vi "TSLIN_Trace monitoring.vi"(10 "Data":T1={"Communication message"={"Sender"="", "receiver"="", "message"="", "data"=variant}, "LIN_Data"={"DLL_PATH"=path "", "Channels used"=1, "Funtiontype"=0, "Rx/TX"=enum."Rx", "Read message type"=enum."Receive&send messages", "async&sync"=enum."async", "sync_sendTimeout"=0, "LIN_SendHead"={"ALINIdxchn"=0, "ALINId"=0, "ALINDLC"=0}, "LIN_Set"={"Hardware Type"=2, "Hardware Subtype"=enum."TC1016", "AHwChannel"=0, "AAppChannel"=19, "ABaudrateKbps"=19.2, "AProtocol"=2, "AldHW"=0}, "LIN_DATA"={"Data0"=0, "Data1"=0, "Data2"=0, "Data3"=0, "Data4"=0, "Data5"=0, "Data6"=0, "Data7"=0}, "LIN_Set_Array"=[], "LDF"={"LDF Path"=path "", "LDF loading channel"=0}, "Blf_Log"={"Blf_Log_PATH"=path ""}, "LIN Scheduling Table Array"=[], "REC_Channel"=0}, "LIN Data array"=[], "error in"={"status"=FALSE, "code"=0, "source"=""}, "REC_Channel"=0, "AsynCall?"=FALSE, "DataBase_array"=refnum} {"REC_Channel" items=["CHN1", "CHN2", "CHN3", "CHN4", "CHN5", "CHN6", "CHN7", "CHN8", "CHN9", "CHN10", "CHN11", "CHN12", "CHN13", "CHN14", "CHN15", "CHN16", "CHN17", "CHN18", "CHN19", "CHN20", "CHN21", "CHN22", "CHN23", "CHN24", "CHN25", "CHN26", "CHN27", "CHN28", "CHN29", "CHN30", "CHN31", "CHN32"]; "LIN_Data"."REC_Channel" items=["CHN1", "CHN2", "CHN3", "CHN4", "CHN5", "CHN6", "CHN7", "CHN8", "CHN9", "CHN10", "CHN11", "CHN12", "CHN13", "CHN14", "CHN15", "CHN16", "CHN17", "CHN18", "CHN19", "CHN20", "CHN21", "CHN22", "CHN23", "CHN24", "CHN25", "CHN26", "CHN27", "CHN28", "CHN29", "CHN30", "CHN31", "CHN32"]; "LIN_Data"."LIN Scheduling Table Array"."LIN_Transmit"."Channel" items=["CHN1", "CHN2", "CHN3", "CHN4", "CHN5", "CHN6", "CHN7", "CHN8", "CHN9", "CHN10", "CHN11", "CHN12", "CHN13", "CHN14", "CHN15", "CHN16", "CHN17", "CHN18", "CHN19", "CHN20", "CHN21", "CHN22", "CHN23", "CHN24", "CHN25", "CHN26", "CHN27", "CHN28", "CHN29", "CHN30", "CHN31", "CHN32"]; "LIN_Data"."LIN Scheduling Table Array"."LIN_Transmit"."ID" format="%.0x"; "LIN_Data"."LIN Scheduling Table Array"."LIN_Transmit"."DLC" format="%.0x"; "LIN_Data"."LIN Scheduling Table Array"."LIN_Transmit"."Set_node_funtiontype" items=["MasterNode", "SlaveNode", "MonitorNote"]; "LIN_Data"."LDF"."LDF loading channel" items=["CHN1", "CHN2", "CHN3", "CHN4", "CHN5", "CHN6", "CHN7", "CHN8", "CHN9", "CHN10", "CHN11", "CHN12", "CHN13", "CHN14", "CHN15", "CHN16", "CHN17", "CHN18", "CHN19", "CHN20", "CHN21", "CHN22", "CHN23", "CHN24", "CHN25", "CHN26", "CHN27", "CHN28", "CHN29", "CHN30", "CHN31", "CHN32"]; "LIN_Data"."LIN_Set_Array"."Set_node_funtiontype" items=["MasterNode", "SlaveNode", "MonitorNote"]; "LIN_Data"."LIN_Set_Array"."Set"."Hardware Type" items=["BUS_UNKNOWN_TYPE", "TS_TCP_DEVICE", "XL_USB_DEVICE", "TS_USB_DEVICE", "PEAK_USB_DEVICE", "KVASER_USB_DEVICE", "ZLG_USB_DEVICE", "ICS_USB_DEVICE", "TS_TC1005_DEVICE", "CANABLE_USB_DEVICE", "TS_WIRELESS_OBD", "TS_USB_DEVICE_EX", "IXXAT_USB_DEVICE", "TS_ETH_IF_DEVICE", "TS_USB_IF_DEVICE", "BUS_DEV_TYPE_COUNT"]; "LIN_Data"."LIN_Set_Array"."Set"."AHwChannel" items=["CHN1", "CHN2", "CHN3", "CHN4", "CHN5", "CHN6", "CHN7", "CHN8", "CHN9", "CHN10", "CHN11", "CHN12", "CHN13", "CHN14", "CHN15", "CHN16", "CHN17", "CHN18", "CHN19", "CHN20", "CHN21", "CHN22", "CHN23", "CHN24", "CHN25", "CHN26", "CHN27", "CHN28", "CHN29", "CHN30", "CHN31", "CHN32"]; "LIN_Data"."LIN_Set_Array"."Set"."AAppChannel" items=["CHN1", "CHN2", "CHN3", "CHN4", "CHN5", "CHN6", "CHN7", "CHN8", "CHN9", "CHN10", "CHN11", "CHN12", "CHN13", "CHN14", "CHN15", "CHN16", "CHN17", "CHN18", "CHN19", "CHN20", "CHN21", "CHN22", "CHN23", "CHN24", "CHN25", "CHN26", "CHN27", "CHN28", "CHN29", "CHN30", "CHN31", "CHN32"]; "LIN_Data"."LIN_Set_Array"."Set"."AProtocol" items=["Lin_Protocol_13", "Lin_Protocol_20", "Lin_Protocol_21", "Lin_Protocol_J2602"]; "LIN_Data"."Funtiontype" items=["MasterNode", "SlaveNode", "MonitorNote"]; "LIN_Data"."LIN_SendHead"."ALINDLC" format="%.0x"; "LIN_Data"."LIN_SendHead"."ALINId" format="%.0x"; "LIN_Data"."LIN_SendHead"."ALINIdxchn" items=["CHN1", "CHN2", "CHN3", "CHN4", "CHN5", "CHN6", "CHN7", "CHN8", "CHN9", "CHN10", "CHN11", "CHN12", "CHN13", "CHN14", "CHN15", "CHN16", "CHN17", "CHN18", "CHN19", "CHN20", "CHN21", "CHN22", "CHN23", "CHN24", "CHN25", "CHN26", "CHN27", "CHN28", "CHN29", "CHN30", "CHN31", "CHN32"]; "LIN_Data"."LIN_Set"."Hardware Type" items=["BUS_UNKNOWN_TYPE", "TS_TCP_DEVICE", "XL_USB_DEVICE", "TS_USB_DEVICE", "PEAK_USB_DEVICE", "KVASER_USB_DEVICE", "ZLG_USB_DEVICE", "ICS_USB_DEVICE", "TS_TC1005_DEVICE", "CANABLE_USB_DEVICE", "TS_WIRELESS_OBD", "TS_USB_DEVICE_EX", "IXXAT_USB_DEVICE", "TS_ETH_IF_DEVICE", "TS_USB_IF_DEVICE", "BUS_DEV_TYPE_COUNT"]; "LIN_Data"."LIN_Set"."AHwChannel" items=["CHN1", "CHN2", "CHN3", "CHN4", "CHN5", "CHN6", "CHN7", "CHN8", "CHN9", "CHN10", "CHN11", "CHN12", "CHN13", "CHN14", "CHN15", "CHN16", "CHN17", "CHN18", "CHN19", "CHN20", "CHN21", "CHN22", "CHN23", "CHN24", "CHN25", "CHN26", "CHN27", "CHN28", "CHN29", "CHN30", "CHN31", "CHN32"]; "LIN_Data"."LIN_Set"."AAppChannel" items=["CHN1", "CHN2", "CHN3", "CHN4", "CHN5", "CHN6", "CHN7", "CHN8", "CHN9", "CHN10", "CHN11", "CHN12", "CHN13", "CHN14", "CHN15", "CHN16", "CHN17", "CHN18", "CHN19", "CHN20", "CHN21", "CHN22", "CHN23", "CHN24", "CHN25", "CHN26", "CHN27", "CHN28", "CHN29", "CHN30", "CHN31", "CHN32"]; "LIN_Data"."LIN_Set"."AProtocol" items=["Lin_Protocol_13", "Lin_Protocol_20", "Lin_Protocol_21", "Lin_Protocol_J2602"]; "LIN_Data"."Channels used" items=["1 Channel"=1, "2 Channels"=2, "3 Channels"=3, "4 Channels"=4, "5 Channels"=5]}, 11 "Sender":string) -> ()   [LabVIEW 2014]
uses:
  Utilities/Typedef/Hardware_Subtype.ctl
  Typedef/TSLIN_SetData.ctl
  Typedef/TSLIN_SendHead.ctl
  Typedef/TSLIN_Config.ctl
  Typedef/TLibLIN.ctl
  Typedef/TSLIN_Data.ctl
  Typedef/TSLIN_Transmit.ctl
  Typedef/TSLIN_LIN Schedule_Table.ctl
  Typedef/TSLIN_LIN_Set.ctl
  All_Control/Typedef/Hardware Type.ctl
  All_Control/Typedef/Blf_Log.ctl
  DataBase/Typedef/CAN/TCANSignal.ctl
  DataBase/Typedef/LIN/TLINSignal.ctl
  DataBase/Typedef/FlexRay/TFlexRaySignal.ctl
  DataBase/Typedef/TDBSignalProperties.ctl
  DataBase/Typedef/TDBFrameProperties.ctl
  DataBase/Typedef/TDBECUProperties.ctl
  DataBase/Typedef/TDBProperties.ctl
  DataBase/Typedef/DataBase_array.ctl
  DataBase/Typedef/DataBase_array_index.ctl
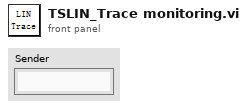
[diagram p1: front panel]
types:
  T1 = typedef "TSLIN_Data.ctl" = cluster{"Communication message":cluster{"Sender":string, "receiver":string, "message":string, "data":variant}, "LIN_Data":T2, "LIN Data array":T11[], "error in":errorcluster, "REC_Channel":i32, "AsynCall?":bool, "DataBase_array":T12}
  T2 = typedef "TSLIN_Config.ctl" = cluster{"DLL_PATH":path, "Channels used":u16, "Funtiontype":i32, "Rx/TX":enum16{"Rx", "Tx"}, "Read message type":enum16{"Only read received messages", "Receive&send messages"}, "async&sync":enum16{"async", "sync"}, "sync_sendTimeout":u16, "LIN_SendHead":T3, "LIN_Set":T4, "LIN_DATA":cluster{"Data0":u8, "Data1":u8, "Data2":u8, "Data3":u8, "Data4":u8, "Data5":u8, "Data6":u8, "Data7":u8}, "LIN_Set_Array":T7[], "LDF":cluster{"LDF Path":path, "LDF loading channel":i32}, "Blf_Log":T8, "LIN Scheduling Table Array":T9[], "REC_Channel":i32}
  T3 = typedef "TSLIN_SendHead.ctl" = cluster{"ALINIdxchn":u8, "ALINId":u32, "ALINDLC":u32}
  T4 = typedef "TSLIN_SetData.ctl" = cluster{"Hardware Type":T5, "Hardware Subtype":T6, "AHwChannel":i32, "AAppChannel":i32, "ABaudrateKbps":sgl, "AProtocol":i32, "AldHW":i32}
  T5 = typedef "Hardware Type.ctl" = i32
  T6 = typedef "Hardware_Subtype.ctl" = enum16{"TS_UNKNOWN_DEVICE", "TSCAN_PRO", "TSCAN_Lite1", "TC1001", "TL1001", "TC1011", "TM5011", "TC1002", "TC1014", "TSCANFD2517", "TC1026", "TC1016", "TC1012", "TC1013", "TLog1002", "TC1034", "TC1018", "GW2116", "TC2115", "MP1013", "TC1113", "TC1114", "TP1013", "TC1017", "TP1018", "TF10XX", "TL1004_FD_4_LIN_2", "TE1051", "TP1051", "TP1034", "TTS9015", "TP1026", "TTS1026", "TTS1034", "TTS1018", "TL1011", "TTS1015_LiAuto", "TTS1013_LiAuto", "TTS1016Pro", "TC1054Pro", "TC1054", "TLog1038", "TO1013", "TC1034Pro", "TC1018Pro", "TC1038Pro", "TS_DEV_END"}
  T7 = typedef "TSLIN_LIN_Set.ctl" = cluster{"Set":T4, "Set_node_funtiontype":i32}
  T8 = typedef "Blf_Log.ctl" = cluster{"Blf_Log_PATH":path}
  T9 = typedef "TSLIN_LIN Schedule_Table.ctl" = cluster{"LIN_Transmit":T10, "Delay(ms)":i32}
  T10 = typedef "TSLIN_Transmit.ctl" = cluster{"Channel":i32, "Rx/TX":enum16{"Rx", "Tx"}, "Set_node_funtiontype":i32, "DLC":u32, "ID":u32, "FDatas":cluster{"value0":u8, "value 1":u8, "value 2":u8, "value 3":u8, "value 4":u8, "value 5":u8, "value 6":u8, "value 7":u8}}
  T11 = typedef "TLibLIN.ctl" = cluster{"Ch":u8, "Code":u8, "Properties":u8, "FDLC":u8, "ID":u8, "Checksum":u8, "FStaus":u8, "FTimeUS":u64, "FDatas":cluster{"value0":u8, "value 1":u8, "value 2":u8, "value 3":u8, "value 4":u8, "value 5":u8, "value 6":u8, "value 7":u8}}
  T12 = typedef "DataBase_array_index.ctl" = refnum<vi>
  T13 = cluster{"Sender":string, "receiver":string, "message":string, "data":variant}
  T14 = enum32{"invalid app kind", "Development System", "Run Time System", "Student Edition", "Embedded LabVIEW", "Evaluation", "Custom"}
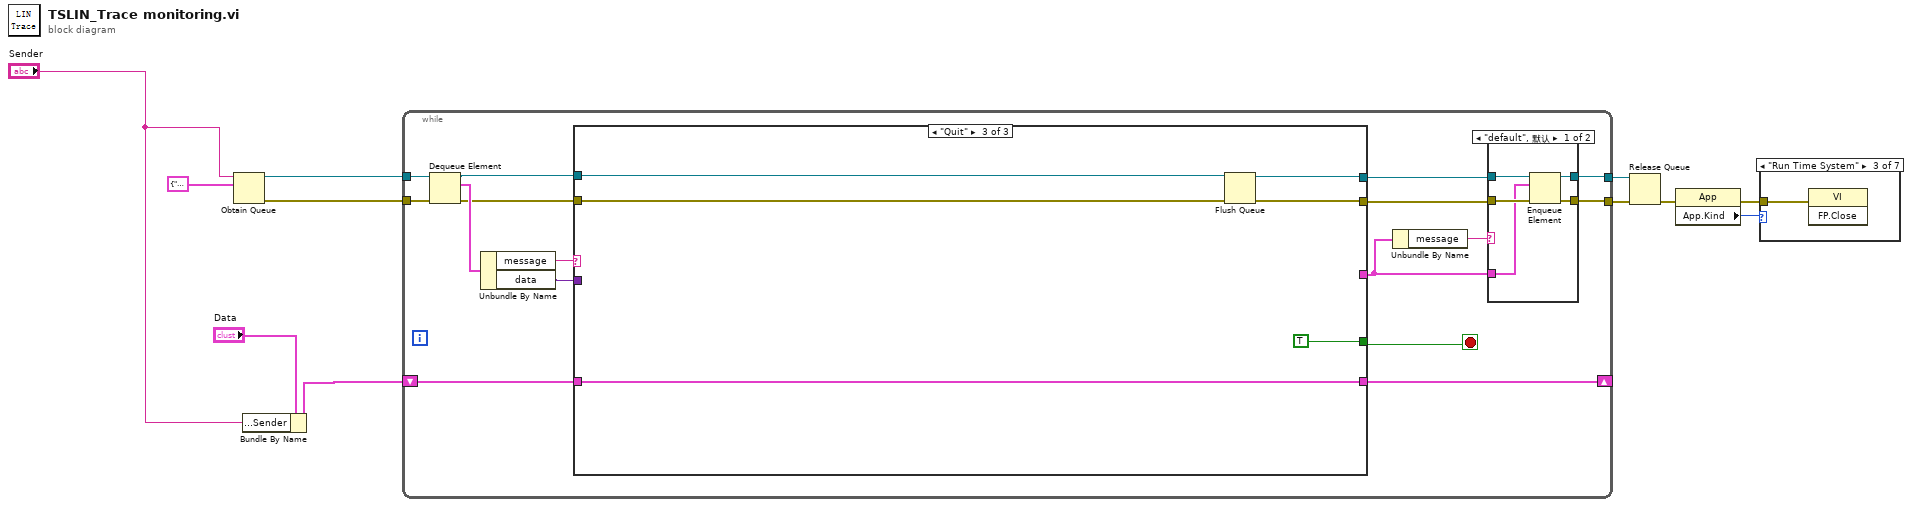
[diagram p0: block diagram]
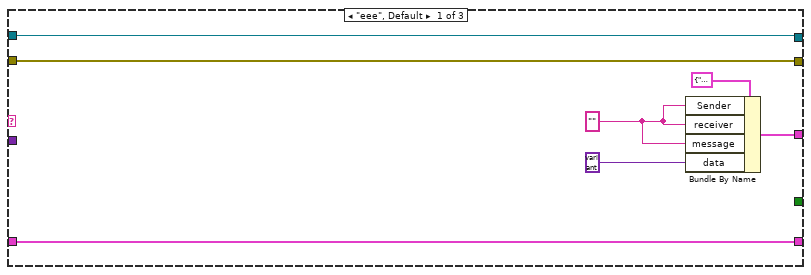
[diagram p9: hidden frame]
diagram:
  n1 = Obtain Queue(name (unnamed)="Sender", element data type=T13 {"Sender"="", "receiver"="", "message"="", "data"=variant} ("Communication message")) -> (queue out=w11:refnum<queue>, error out=w4:errorcluster)  [unwired: 3 in, 1 out]
  n2 = Bundle By Name(cluster="Data", "Communication message.Sender"="Sender") -> (w2:T1)
  n3 = while {
    tunnel: w11 -> [w27]
    tunnel: w4 -> [w26]
    tunnel: [w18] -> w10
    tunnel: [w17] -> w9
    shift-right: [w12] -> _
    shift-left: w2 -> [w13]
    stop <- w16 stop-if-true
    n4 = Dequeue Element(queue=w27, error in (no error)=w26) -> (queue out=w23:refnum<queue>, element=w25:T13, error out=w22:errorcluster)  [unwired: 1 in, 1 out]
    n5 = Unbundle By Name(w25) -> ("message"=w24:string, "data"=w19:variant)
    n6 = case shown="\"Quit\"" w24 {
      tunnel: [w41 w44 w49] -> w21
      tunnel: w23 -> [w41 w44 w48]
      tunnel: w22 -> [w40 w43 w46]
      tunnel: [w40 w43 w47] -> w20
      tunnel: w19 -> [_ _ _]
      tunnel: [_ _ TRUE] -> w16
      tunnel: [w38 _ _] -> w15
      tunnel: [w35 w42 w45] -> w12
      tunnel: w13 -> [w35 w42 w45]
      frame "eee", Default {
        w36 = ""
        n7 = Bundle By Name(cluster=T13 {"Sender"="", "receiver"="", "message"="", "data"=variant} ("Communication message"), "Sender"=w36, "receiver"=w36, "message"=w36, "data"=variant) -> (w38:T13)
      }
      frame "Init" {
      }
      frame "Quit" {
        n8 = Flush Queue(queue=w48, error in (no error)=w46) -> (queue out=w49:refnum<queue>, error out=w47:errorcluster)  [unwired: 1 out]
      }
    }
    n9 = Unbundle By Name(w15) -> ("message"=w14:string)
    n10 = case shown="\"default\", 默认" w14 {
      tunnel: w21 -> [w32 w34]
      tunnel: w20 -> [w31 w33]
      tunnel: w15 -> [w30 _]
      tunnel: [w29 w34] -> w18
      tunnel: [w28 w33] -> w17
      frame "default", Default {
        n11 = Enqueue Element(queue=w32, element=w30, error in (no error)=w31) -> (queue out=w29:refnum<queue>, error out=w28:errorcluster)  [unwired: 1 in, 1 out]
      }
      frame "" {
      }
    }
  }
  n12 = Release Queue(queue=w10, error in (no error)=w9) -> (error out=w8:errorcluster)  [unwired: 1 in, 2 out]
  n13 = property class="App"(error in=w8) -> (error out=w7:errorcluster, "App.Kind"=w6:T14)  [unwired: 1 in, 1 out]
  n14 = case shown="\"Run Time System\"" w6 {
    tunnel: w7 -> [_ _ w51 _ _ _ _]
    frame "invalid app kind", Default {
    }
    frame "Development System" {
    }
    frame "Run Time System" {
      n15 = invoke class="VI" method="FP.Close"(error in=w51) -> ()  [unwired: 2 in, 3 out]
    }
    frame "Student Edition" {
    }
    frame "Embedded LabVIEW" {
    }
    frame "Evaluation" {
    }
    frame "Custom" {
    }
  }
